vi "Periodic Tasks.vi"() -> ()   [LabVIEW 2019]
doc: "This VI runs in parallel to other tasks. It can contain as many user-defined periodic loops as you need. These can carry out PID or other sorts of timed response."
uses:
  <vilib>/Rock Robotics/WPI/Utilities/WPI_GetSetVariantRefNum.vi
  <vilib>/Utility/config.llb/Read Key (Double).vi
  <vilib>/Utility/config.llb/NI_LVConfig.lvlib
panel:
  out "TRUE 3":bool
  out "Loop Count 2":i32
  out "Numeric 2":i32
  out "Scaler":i8=127
  out "Normalized Color 2":cluster{"R":dbl, "G":dbl, "B":dbl}
  out "element 3":bool
  out "Color Match Name":string
  out "TRUE 1":bool
  out "TRUE 2":bool
  out "Numeric":i32
  out "Color is matched":bool
  out "element 2":bool
  out "Loop Count":i32
  out "element":bool
  out "Matched Color Name":string
  out "Confidence":dbl
  out "Matched Color":cluster{"R":dbl, "G":dbl, "B":dbl}
  out "Color":u32(colorbox)
  out "Normalized Color":cluster{"R":dbl, "G":dbl, "B":dbl}
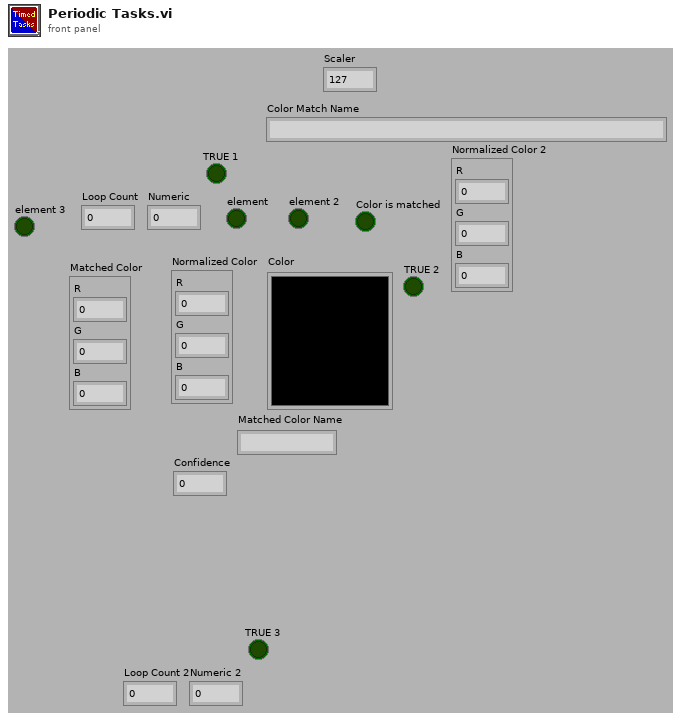
[diagram p1: front panel]
types:
  T1 = typedef "NI_LVConfig.lvlib/Config Data RefNum.ctl" = refnum<k1>
  T2 = typedef "WPI_JoystickDevRef.ctl" = cluster{"Device":T3}
  T3 = typedef "WPI_JoystickDeviceEnum.ctl" = enum16{"USB 0", "USB 1", "USB 2", "USB 3", "USB 4", "USB 5"}
  T4 = typedef "Color Sensor V3 DevRef.ctl" = cluster{"I2CDevRef":T5}
  T5 = typedef "WPI_I2CDevRef.ctl" = cluster{"DevStatus":errorcluster, "Device Address":u8, "Handle":i32, "I2C Bus":T6}
  T6 = typedef "i2c_bus.ctl" = enum16{"I2C On-Board", "I2C MXP", "Invalid"}
  T7 = typedef "WPI_MotorControlDeviceRef.ctl" = cluster{"DeviceStatus":errorcluster, "Type":T8, "PWM":cluster{"PWM Channel":T9, "DeadBand":T10}, "CAN":cluster{"Device Number":u8, "SetOutput VI Ref":variant, "GetOutput VI Ref":variant, "Enable VI Ref":variant, "Disable VI Ref":variant, "Data":variant}, "Invert":bool, "DIO PWM":cluster{"PWM \"Enable\" Channel":T9, "DIOChannel":T11, "PWM Rate":dbl}}
  T8 = typedef "WPI_MotorControlType.ctl" = enum16{"PWM", "CAN", "DIO PWM"}
  T9 = typedef "FPGA_DIOPWMChannel.ctl" = enum8{"PWM 0", "PWM 1", "PWM 2", "PWM 3", "PWM 4", "PWM 5", "PWM 6", "PWM 7", "PWM 8", "PWM 9", "PWM MXP 0", "PWM MXP 1", "PWM MXP 2", "PWM MXP 3", "PWM MXP 4", "PWM MXP 5", "PWM MXP 6", "PWM MXP 7", "PWM MXP 8", "PWM MXP 9", "Invalid"}
  T10 = typedef "WPI_PWMDeadband.ctl" = cluster{"Name":string, "maxPositivePwm":i32, "minPositivePwm":i32, "centerPwm":i32, "maxNegativePwm":i32, "minNegativePwm":i32, "angularRange":u16}
  T11 = typedef "FPGA_DIOChannel.ctl" = enum8{"DIO 0", "DIO 1", "DIO 2", "DIO 3", "DIO 4", "DIO 5", "DIO 6", "DIO 7", "DIO 8", "DIO 9", "DIO MXP 0", "DIO MXP 1", "DIO MXP 2", "DIO MXP 3", "DIO MXP 4", "DIO MXP 5", "DIO MXP 6", "DIO MXP 7", "DIO MXP 8", "DIO MXP 9", "DIO MXP 10", "DIO MXP 11", "DIO MXP 12", "DIO MXP 13", "DIO MXP 14", "DIO MXP 15", "SPI Port CS1", "SPI Port CS2", "SPI Port CS3", "SPI Port MISO", "SPI Port MOSI", "Invalid"}
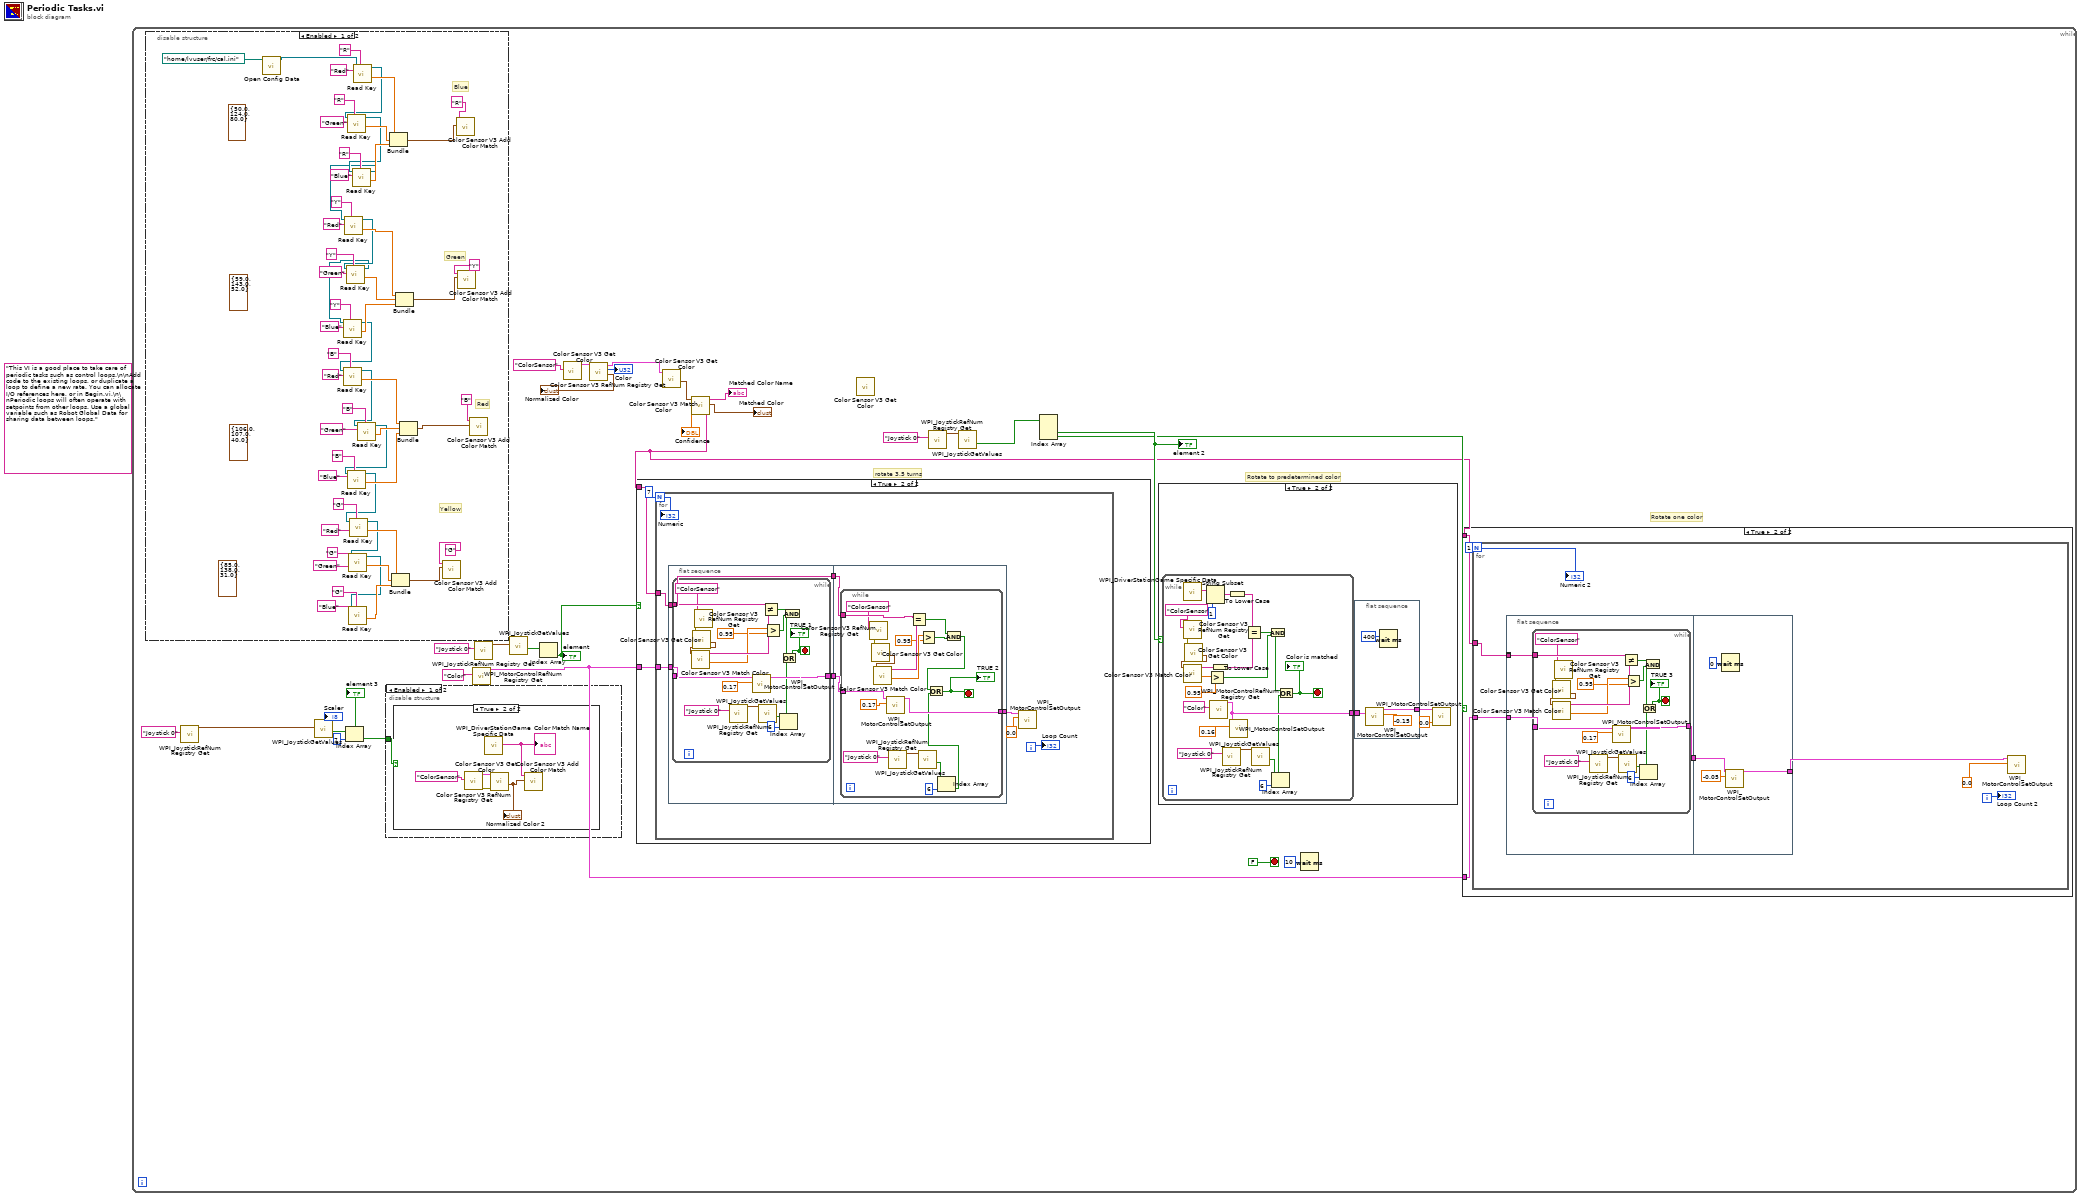
[diagram p0: block diagram]
diagram:
  (unwired) "This VI is a good place to take care of periodic tasks such as control loops.\n\nAdd code to the existing loops, or duplicate a loop to define a new rate. You can allocate I/O references here, or in Begin.vi.\n\nPeriodic loops will often operate with setpoints from other loops. Use a global variable such as Robot Global Data for sharing data between loops."
  n1 = while {
    stop <- FALSE stop-if-true
    # "rotate 3.5 turns"
    # "Rotate to predetermined color"
    # "Rotate one color"
    n2 = disable-structure shown="Enabled" {
      frame Enabled {
        (unwired) cluster{"R":dbl, "G":dbl, "B":dbl} {"R"=85.0, "G"=138.0, "B"=31.0} ("Color")
        (unwired) cluster{"R":dbl, "G":dbl, "B":dbl} {"R"=106.0, "G"=107.0, "B"=40.0} ("Color")
        (unwired) cluster{"R":dbl, "G":dbl, "B":dbl} {"R"=59.0, "G"=143.0, "B"=52.0} ("Color")
        (unwired) cluster{"R":dbl, "G":dbl, "B":dbl} {"R"=50.0, "G"=124.0, "B"=80.0} ("Color")
        # "Red"
        # "Green"
        # "Yellow"
        # "Blue"
        n3 = call <vilib>:"Open Config Data.vi"("configuration file path"=path "/home/lvuser/frc/cal.ini") -> ("refnum"=w72:T1)  [unwired: 8 in, 2 out]
        n4 = call-poly <vilib>:"Read Key.vi"("section"="R", "key"="Red", "refnum"=w72) -> ("value"=w97:dbl, "refnum out"=w96:T1)  [unwired: 5 in, 2 out]
        n5 = call-poly <vilib>:"Read Key.vi"("section"="R", "key"="Green", "refnum"=w96) -> ("value"=w98:dbl, "refnum out"=w95:T1)  [unwired: 5 in, 2 out]
        n6 = call-poly <vilib>:"Read Key.vi"("section"="R", "key"="Blue", "refnum"=w95) -> ("value"=w99:dbl, "refnum out"=w94:T1)  [unwired: 5 in, 2 out]
        n7 = call-poly <vilib>:"Read Key.vi"("section"="Y", "key"="Red", "refnum"=w94) -> ("value"=w93:dbl, "refnum out"=w80:T1)  [unwired: 5 in, 2 out]
        n8 = call-poly <vilib>:"Read Key.vi"("section"="Y", "key"="Green", "refnum"=w80) -> ("value"=w92:dbl, "refnum out"=w79:T1)  [unwired: 5 in, 2 out]
        n9 = call-poly <vilib>:"Read Key.vi"("section"="Y", "key"="Blue", "refnum"=w79) -> ("value"=w91:dbl, "refnum out"=w78:T1)  [unwired: 5 in, 2 out]
        n10 = call-poly <vilib>:"Read Key.vi"("section"="B", "key"="Red", "refnum"=w78) -> ("value"=w85:dbl, "refnum out"=w77:T1)  [unwired: 5 in, 2 out]
        n11 = call-poly <vilib>:"Read Key.vi"("section"="B", "key"="Green", "refnum"=w77) -> ("value"=w87:dbl, "refnum out"=w76:T1)  [unwired: 5 in, 2 out]
        n12 = call-poly <vilib>:"Read Key.vi"("section"="B", "key"="Blue", "refnum"=w76) -> ("value"=w86:dbl, "refnum out"=w75:T1)  [unwired: 5 in, 2 out]
        n13 = call-poly <vilib>:"Read Key.vi"("section"="G", "key"="Red", "refnum"=w75) -> ("value"=w88:dbl, "refnum out"=w74:T1)  [unwired: 5 in, 2 out]
        n14 = call-poly <vilib>:"Read Key.vi"("section"="G", "key"="Green", "refnum"=w74) -> ("value"=w89:dbl, "refnum out"=w73:T1)  [unwired: 5 in, 2 out]
        n15 = call-poly <vilib>:"Read Key.vi"("section"="G", "key"="Blue", "refnum"=w73) -> ("value"=w90:dbl)  [unwired: 5 in, 3 out]
        n16 = Bundle("value"=w97, "value"=w98, "value"=w99) -> (w81:cluster{"value":dbl, "value":dbl, "value":dbl})  [unwired: 1 in]
        n17 = Bundle("value"=w88, "value"=w89, "value"=w90) -> (w83:cluster{"value":dbl, "value":dbl, "value":dbl})  [unwired: 1 in]
        n18 = Bundle("value"=w93, "value"=w92, "value"=w91) -> (w82:cluster{"value":dbl, "value":dbl, "value":dbl})  [unwired: 1 in]
        n19 = Bundle("value"=w85, "value"=w87, "value"=w86) -> (w84:cluster{"value":dbl, "value":dbl, "value":dbl})  [unwired: 1 in]
        n20 = call <vilib>:"Color Sensor V3 Add Color Match.vi"("Color"=w83, "Name"="G") -> ()  [unwired: 10 in]
        n21 = call <vilib>:"Color Sensor V3 Add Color Match.vi"("Color"=w81, "Name"="R") -> ()  [unwired: 10 in]
        n22 = call <vilib>:"Color Sensor V3 Add Color Match.vi"("Color"=w82, "Name"="Y") -> ()  [unwired: 10 in]
        n23 = call <vilib>:"Color Sensor V3 Add Color Match.vi"("Color"=w84, "Name"="B") -> ()  [unwired: 10 in]
      }
      frame Disabled {
      }
    }
    n24 = call <vilib>:"WPI_JoystickRefNum Registry Get.vi"("refnum name"="Joystick 0") -> ("JoystickDevRef"=w8:T2)  [unwired: 9 in, 1 out]
    n25 = call <vilib>:"WPI_JoystickGetValues.vi"("JoystickDevRef"=w8) -> ("Buttons"=w10:bool[])  [unwired: 6 in, 4 out]
    n26 = Index Array(array=w10, index=7) -> (element=w7:bool)
    "element 3" <- w7
    n27 = disable-structure shown="Enabled" {
      disable-tunnel: w7 -> [w65 _]
      frame Enabled {
        n28 = case shown="True" w65 {
          frame False {
          }
          frame True {
            n29 = call <vilib>:"Color Sensor V3 RefNum Registry Get.vi"("refnum name"="ColorSensor") -> ("error out"=w69:errorcluster, "ColorSensorDevRef"=w67:T4)  [unwired: 9 in]
            n30 = call <vilib>:"WPI_DriverStationGame Specific Data.vi"() -> ("Game Specific Data"=w70:string)  [unwired: 11 in]
            "Color Match Name" <- w70
            n31 = call <vilib>:"Color Sensor V3 Get Color.vi"("error in (no error)"=w69, "ColorSensorDevRef"=w67) -> ("Normalized Color"=w68:cluster{"R":dbl, "G":dbl, "B":dbl})  [unwired: 6 in, 3 out]
            "Normalized Color 2" <- w68
            n32 = call <vilib>:"Color Sensor V3 Add Color Match.vi"("Color"=w68, "Name"=w70) -> ()  [unwired: 10 in]
          }
        }
      }
      frame Disabled {
      }
    }
    n33 = call <vilib>:"WPI_MotorControlRefNum Registry Get.vi"("refnum name"="Color") -> ("MotorControlDevRef"=w2:T7)  [unwired: 9 in, 1 out]
    n34 = call <vilib>:"WPI_JoystickRefNum Registry Get.vi"("refnum name"="Joystick 0") -> ("JoystickDevRef"=w18:T2)  [unwired: 9 in, 1 out]
    n35 = call <vilib>:"WPI_JoystickGetValues.vi"("JoystickDevRef"=w18) -> ("Buttons"=w17:bool[])  [unwired: 6 in, 4 out]
    n36 = Index Array(array=w17) -> (element=w12:bool)  [unwired: 1 in]
    "element" <- w12
    n37 = call <vilib>:"Color Sensor V3 RefNum Registry Get.vi"("refnum name"="ColorSensor") -> ("ColorSensorDevRef"=w25:T4)  [unwired: 9 in, 1 out]
    n38 = call <vilib>:"Color Sensor V3 Get Color.vi"("ColorSensorDevRef"=w25) -> ("Normalized Color"=→"Normalized Color":cluster{"R":dbl, "G":dbl, "B":dbl}, "Color"=→"Color":u32, "ColorSensorDevRef out"=w4:T4)  [unwired: 7 in, 1 out]
    n39 = call <vilib>:"Color Sensor V3 Get Color.vi"("ColorSensorDevRef"=w4) -> ("Normalized Color"=w20:cluster{"R":dbl, "G":dbl, "B":dbl})  [unwired: 7 in, 3 out]
    n40 = call <vilib>:"Color Sensor V3 Match Color.vi"("Measured Color"=w20) -> ("Confidence"=→"Confidence":dbl, "Matched Color"=→"Matched Color":cluster{"R":dbl, "G":dbl, "B":dbl}, "Matched Color Name"=w1:string)  [unwired: 8 in]
    "Matched Color Name" <- w1
    n41 = case shown="True" w12 {
      tunnel: w1 -> [_ w161]
      tunnel: w2 -> [_ w160]
      frame False {
      }
      frame True {
        n42 = for {
          N: 7 -> [w164]
          tunnel: w161 -> [w167]
          tunnel: w160 -> [w166]
          i -> [w165]
          n43 = flat-sequence {
            tunnel: [w171] -> _
            tunnel: w167 -> [w171]
            tunnel: w166 -> [w172]
            tunnel: [w170] -> w169
            tunnel: [w171] -> w168
            tunnel: w169 -> [w194]
            tunnel: w168 -> [w195]
            tunnel: [w193] -> w162
            frame #0 {
              n44 = while {
                tunnel: w171 -> [w189]
                tunnel: w172 -> [w192]
                tunnel: [w181] -> w170
                stop <- w177 stop-if-true
                n45 = call <vilib>:"Color Sensor V3 RefNum Registry Get.vi"("refnum name"="ColorSensor") -> ("error out"=w188:errorcluster, "ColorSensorDevRef"=w187:T4)  [unwired: 9 in]
                n46 = call <vilib>:"Color Sensor V3 Get Color.vi"("error in (no error)"=w188, "ColorSensorDevRef"=w187) -> ("Normalized Color"=w186:cluster{"R":dbl, "G":dbl, "B":dbl})  [unwired: 6 in, 3 out]
                n47 = call <vilib>:"Color Sensor V3 Match Color.vi"("Measured Color"=w186) -> ("Confidence"=w184:dbl, "Matched Color Name"=w191:string)  [unwired: 8 in, 1 out]
                n48 = call <vilib>:"WPI_JoystickRefNum Registry Get.vi"("refnum name"="Joystick 0") -> ("JoystickDevRef"=w179:T2)  [unwired: 9 in, 1 out]
                n49 = call <vilib>:"WPI_MotorControlSetOutput.vi"("Output"=0.17 ("Motor Output"), "MotorControlDevRef"=w192) -> ("MotorControlDevRef"=w181:T7)  [unwired: 7 in, 2 out]
                n50 = call <vilib>:"WPI_JoystickGetValues.vi"("JoystickDevRef"=w179) -> ("Buttons"=w178:bool[])  [unwired: 6 in, 4 out]
                n51 = Not Equal?(x=w189, y=w191) -> (x != y?=w185:bool)
                n52 = Greater?(x=w184, y=0.95) -> (0:w182:bool)
                n53 = Index Array(array=w178, index=6) -> (element=w176:bool)
                n54 = And(x=w185, y=w182) -> (x .and. y?=w175:bool)
                n55 = Or(x=w175, y=w176) -> (x .or. y?=w177:bool)
                "TRUE 1" <- w177
              }
            }
            frame #1 {
              n56 = while {
                tunnel: w195 -> [w213]
                tunnel: w194 -> [w215]
                tunnel: [w204] -> w193
                stop <- w198 stop-if-true
                n57 = call <vilib>:"Color Sensor V3 RefNum Registry Get.vi"("refnum name"="ColorSensor") -> ("error out"=w212:errorcluster, "ColorSensorDevRef"=w211:T4)  [unwired: 9 in]
                n58 = call <vilib>:"Color Sensor V3 Get Color.vi"("error in (no error)"=w212, "ColorSensorDevRef"=w211) -> ("Normalized Color"=w210:cluster{"R":dbl, "G":dbl, "B":dbl})  [unwired: 6 in, 3 out]
                n59 = call <vilib>:"Color Sensor V3 Match Color.vi"("Measured Color"=w210) -> ("Confidence"=w206:dbl, "Matched Color Name"=w214:string)  [unwired: 8 in, 1 out]
                n60 = call <vilib>:"WPI_MotorControlSetOutput.vi"("Output"=0.17, "MotorControlDevRef"=w215) -> ("MotorControlDevRef"=w204:T7)  [unwired: 7 in, 2 out]
                n61 = call <vilib>:"WPI_JoystickRefNum Registry Get.vi"("refnum name"="Joystick 0") -> ("JoystickDevRef"=w202:T2)  [unwired: 9 in, 1 out]
                n62 = Equal?(x=w213, y=w214) -> (x = y?=w207:bool)
                n63 = call <vilib>:"WPI_JoystickGetValues.vi"("JoystickDevRef"=w202) -> ("Buttons"=w201:bool[])  [unwired: 6 in, 4 out]
                n64 = Greater?(x=w206, y=0.95) -> (0:w208:bool)
                n65 = Index Array(array=w201, index=6) -> (element=w200:bool)
                n66 = And(x=w207, y=w208) -> (x .and. y?=w199:bool)
                n67 = Or(x=w199, y=w200) -> (x .or. y?=w198:bool)
                "TRUE 2" <- w198
              }
            }
          }
          n68 = call <vilib>:"WPI_MotorControlSetOutput.vi"("Output"=0.0, "MotorControlDevRef"=w162) -> ()  [unwired: 7 in, 3 out]
          "Loop Count" <- w165
          "Numeric" <- w164
        }
      }
    }
    n69 = call <vilib>:"Color Sensor V3 Get Color.vi"() -> ()  [unwired: 8 in, 4 out]
    n70 = call <vilib>:"WPI_JoystickRefNum Registry Get.vi"("refnum name"="Joystick 0") -> ("JoystickDevRef"=w15:T2)  [unwired: 9 in, 1 out]
    n71 = call <vilib>:"WPI_JoystickGetValues.vi"("JoystickDevRef"=w15) -> ("Buttons"=w14:bool[])  [unwired: 6 in, 4 out]
    n72 = Index Array(array=w14) -> (element #2=w13:bool, element #3=w3:bool)  [unwired: 3 in, 1 out]
    "element 2" <- w13
    n73 = case shown="True" w13 {
      frame False {
      }
      frame True {
        n74 = while {
          tunnel: [w152] -> w129
          stop <- w137 stop-if-true
          n75 = call <vilib>:"Color Sensor V3 RefNum Registry Get.vi"("refnum name"="ColorSensor") -> ("error out"=w156:errorcluster, "ColorSensorDevRef"=w155:T4)  [unwired: 9 in]
          n76 = call <vilib>:"WPI_DriverStationGame Specific Data.vi"() -> ("Game Specific Data"=w147:string)  [unwired: 11 in]
          n77 = call <vilib>:"Color Sensor V3 Get Color.vi"("error in (no error)"=w156, "ColorSensorDevRef"=w155) -> ("Normalized Color"=w154:cluster{"R":dbl, "G":dbl, "B":dbl})  [unwired: 6 in, 3 out]
          n78 = call <vilib>:"Color Sensor V3 Match Color.vi"("Measured Color"=w154) -> ("Confidence"=w150:dbl, "Matched Color Name"=w158:string)  [unwired: 8 in, 1 out]
          n79 = String Subset(string=w147, length (rest)=1 ("length (rest)")) -> (substring=w144:string)  [unwired: 1 in]
          n80 = Greater?(x=w150, y=0.95) -> (0:w148:bool)
          n81 = call <vilib>:"WPI_MotorControlRefNum Registry Get.vi"("refnum name"="Color") -> ("MotorControlDevRef"=w152:T7)  [unwired: 9 in, 1 out]
          n82 = To Lower Case(string=w158) -> (all lower case string=w146:string)
          n83 = call <vilib>:"WPI_JoystickRefNum Registry Get.vi"("refnum name"="Joystick 0") -> ("JoystickDevRef"=w141:T2)  [unwired: 9 in, 1 out]
          n84 = To Lower Case(string=w144) -> (all lower case string=w145:string)
          n85 = call <vilib>:"WPI_MotorControlSetOutput.vi"("Output"=0.16 ("Motor Output"), "MotorControlDevRef"=w152) -> ()  [unwired: 7 in, 3 out]
          n86 = Equal?(x=w145, y=w146) -> (x = y?=w151:bool)
          n87 = call <vilib>:"WPI_JoystickGetValues.vi"("JoystickDevRef"=w141) -> ("Buttons"=w140:bool[])  [unwired: 6 in, 4 out]
          n88 = And(x=w151, y=w148) -> (x .and. y?=w138:bool)
          n89 = Index Array(array=w140, index=6) -> (element=w139:bool)
          n90 = Or(x=w138, y=w139) -> (x .or. y?=w137:bool)
          "Color is matched" <- w137
        }
        n91 = flat-sequence {
          tunnel: w129 -> [w134]
          tunnel: [w131] -> w128
          frame #0 {
            n92 = call <vilib>:"WPI_MotorControlSetOutput.vi"("Output"=-0.15, "MotorControlDevRef"=w134) -> ("MotorControlDevRef"=w131:T7)  [unwired: 7 in, 2 out]
            n93 = Wait (ms)(milliseconds to wait=u32 400) -> ()  [unwired: 1 out]
          }
        }
        n94 = call <vilib>:"WPI_MotorControlSetOutput.vi"("Output"=0.0, "MotorControlDevRef"=w128) -> ()  [unwired: 7 in, 3 out]
      }
    }
    n95 = Wait (ms)(milliseconds to wait=u32 10) -> ()  [unwired: 1 out]
    n96 = case shown="True" w3 {
      tunnel: w2 -> [_ w29]
      tunnel: w1 -> [_ w28]
      frame False {
      }
      frame True {
        n97 = for {
          N: 1 -> [w34]
          tunnel: w28 -> [w37]
          tunnel: w29 -> [w36]
          i -> [w35]
          n98 = flat-sequence {
            tunnel: [w39] -> _
            tunnel: w37 -> [w39]
            tunnel: w36 -> [w40]
            tunnel: [w38] -> w32
            tunnel: w32 -> [w62]
            tunnel: [w61] -> w31
            frame #0 {
              n99 = while {
                tunnel: w39 -> [w57]
                tunnel: w40 -> [w60]
                tunnel: [w49] -> w38
                stop <- w45 stop-if-true
                n100 = call <vilib>:"Color Sensor V3 RefNum Registry Get.vi"("refnum name"="ColorSensor") -> ("error out"=w56:errorcluster, "ColorSensorDevRef"=w55:T4)  [unwired: 9 in]
                n101 = call <vilib>:"Color Sensor V3 Get Color.vi"("error in (no error)"=w56, "ColorSensorDevRef"=w55) -> ("Normalized Color"=w54:cluster{"R":dbl, "G":dbl, "B":dbl})  [unwired: 6 in, 3 out]
                n102 = call <vilib>:"Color Sensor V3 Match Color.vi"("Measured Color"=w54) -> ("Confidence"=w52:dbl, "Matched Color Name"=w59:string)  [unwired: 8 in, 1 out]
                n103 = call <vilib>:"WPI_JoystickRefNum Registry Get.vi"("refnum name"="Joystick 0") -> ("JoystickDevRef"=w47:T2)  [unwired: 9 in, 1 out]
                n104 = call <vilib>:"WPI_MotorControlSetOutput.vi"("Output"=0.17 ("Motor Output"), "MotorControlDevRef"=w60) -> ("MotorControlDevRef"=w49:T7)  [unwired: 7 in, 2 out]
                n105 = call <vilib>:"WPI_JoystickGetValues.vi"("JoystickDevRef"=w47) -> ("Buttons"=w46:bool[])  [unwired: 6 in, 4 out]
                n106 = Not Equal?(x=w57, y=w59) -> (x != y?=w53:bool)
                n107 = Greater?(x=w52, y=0.95) -> (0:w50:bool)
                n108 = Index Array(array=w46, index=6) -> (element=w44:bool)
                n109 = And(x=w53, y=w50) -> (x .and. y?=w43:bool)
                n110 = Or(x=w43, y=w44) -> (x .or. y?=w45:bool)
                "TRUE 3" <- w45
              }
            }
            frame #1 {
              n111 = Wait (ms)(milliseconds to wait=u32 0) -> ()  [unwired: 1 out]
              n112 = call <vilib>:"WPI_MotorControlSetOutput.vi"("Output"=-0.05, "MotorControlDevRef"=w62) -> ("MotorControlDevRef"=w61:T7)  [unwired: 7 in, 2 out]
            }
          }
          n113 = call <vilib>:"WPI_MotorControlSetOutput.vi"("Output"=0.0, "MotorControlDevRef"=w31) -> ()  [unwired: 7 in, 3 out]
          "Loop Count 2" <- w35
          "Numeric 2" <- w34
        }
      }
    }
  }
